vi "SetImage.vi"(2 "image":T1, 3 "tracker":u64) -> (1 "tracker":u64)   [LabVIEW 2011]
uses:
  <vilib>/vision/Image Controls.llb/IMAQ Image.ctl
  cudatrack-debug.dll
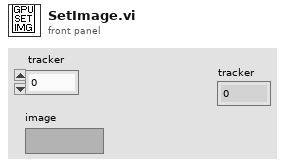
[diagram p1: front panel]
types:
  T1 = typedef "IMAQ Image.ctl" = refnum<image>
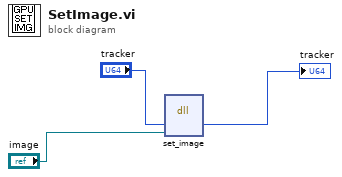
[diagram p0: block diagram]
diagram:
  n1 = dll-call lib="D:/jcnossen1/cudaqi-tracker/cudatrack/cudatrack-debug.dll" fn="set_image"("tracker"="tracker", "image"="image") -> ("tracker"=→"tracker":u64)  [unwired: 5 in, 2 out]
